vi "dev fix timestamp DELETEME.vi"(11 "date time rec":T1) -> (3 "time stamp":timestamp)   [LabVIEW 2018, in "Receipt Parsing.lvlib"]
uses:
  Receipt Parsing.lvlib
  <vilib>/Utility/miscctls.llb/LVDateTimeRec.ctl
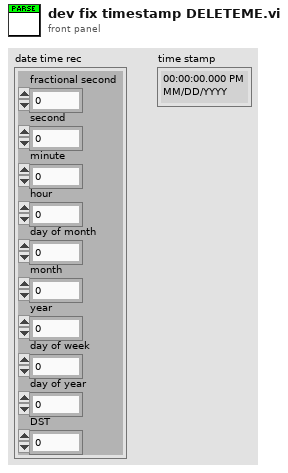
[diagram p1: front panel]
types:
  T1 = typedef "LVDateTimeRec.ctl" = cluster{"fractional second":dbl, "second":i32, "minute":i32, "hour":i32, "day of month":i32, "month":i32, "year":i32, "day of week":i32, "day of year":i32, "DST":i32}
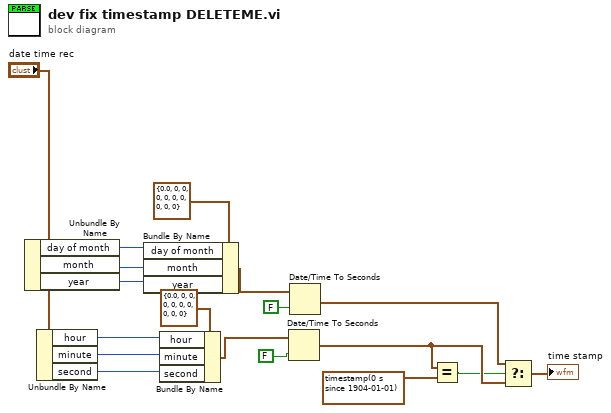
[diagram p0: block diagram]
diagram:
  n1 = Unbundle By Name("date time rec") -> ("day of month"=w1:i32, "month"=w2:i32, "year"=w3:i32)
  n2 = Unbundle By Name("date time rec") -> ("hour"=w5:i32, "minute"=w6:i32, "second"=w7:i32)
  n3 = Bundle By Name(cluster=T1 {"fractional second"=0.0, "second"=0, "minute"=0, "hour"=0, "day of month"=0, "month"=0, "year"=0, "day of week"=0, "day of year"=0, "DST"=0} ("date time rec"), "day of month"=w1, "month"=w2, "year"=w3) -> (w10:T1)
  n4 = Bundle By Name(cluster=T1 {"fractional second"=0.0, "second"=0, "minute"=0, "hour"=0, "day of month"=0, "month"=0, "year"=0, "day of week"=0, "day of year"=0, "DST"=0} ("date time rec"), "hour"=w5, "minute"=w6, "second"=w7) -> (w13:T1)
  n5 = Date/Time To Seconds(1:FALSE ("is UTC (F)"), 2:w13) -> (0:w17:timestamp)
  n6 = Date/Time To Seconds(1:FALSE ("is UTC (F)"), 2:w10) -> (0:w16:timestamp)
  n7 = Equal?(x=w17, y=timestamp(0 s since 1904-01-01) ("time stamp")) -> (x = y?=w15:bool)
  n8 = Select(t=w16, s=w15, f=w17) -> (s? t:f=→"time stamp":timestamp)
